vi "Read Actor Label.vi"(8 "error in (no error)":errorcluster, 11 "Monitored Actor in":refnum<class "Monitored Actor.lvclass">) -> (0 "error out":errorcluster, 2 "Actor Label":string, 3 "Monitored Actor out":refnum<class "Monitored Actor.lvclass">)   [LabVIEW 2017, in "MGI-Monitored Actor Core.lvlib" / "Monitored Actor.lvclass"]
doc: "Reads the Actor's Label.\n----\nCopyright: MGI 2018\nAuthor: Derek Trepanier"
uses:
  Monitored Actor.lvclass
  Monitored Actor.lvclass/Monitored Actor.ctl
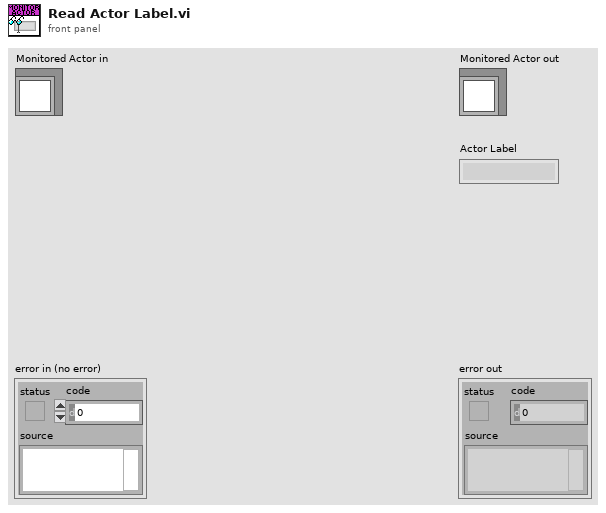
[diagram p1: front panel]
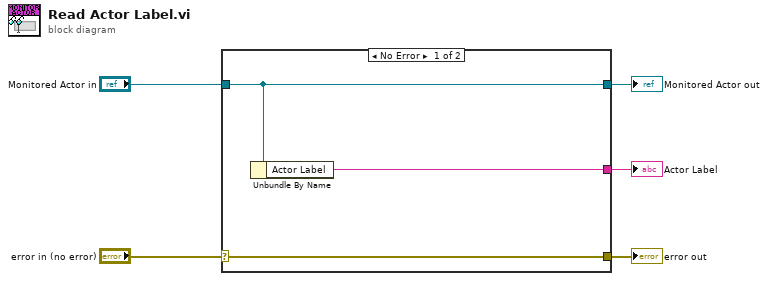
[diagram p0: block diagram]
diagram:
  n1 = case shown="No Error" "error in (no error)" {
    selector: "error in (no error)" -> [w8 w9]
    tunnel: [w8 w9] -> w4
    tunnel: [w7 w10] -> w2
    tunnel: "Monitored Actor in" -> [w7 w10]
    tunnel: [w6 _] -> w1
    frame No Error {
      n2 = Unbundle By Name(w7) -> ("Actor Label"=w6:string)
    }
    frame Error {
    }
  }
  "error out" <- w4
  "Monitored Actor out" <- w2
  "Actor Label" <- w1
